vi "U01_8_5 ReadExcelActiveX.vi"(8 "error in (no error)":errorcluster, 10 "NameSheet":string, 11 "References":T1) -> (0 "error out":errorcluster, 2 "data":string[][](array[string]), 3 "References":T1)   [LabVIEW 2019]
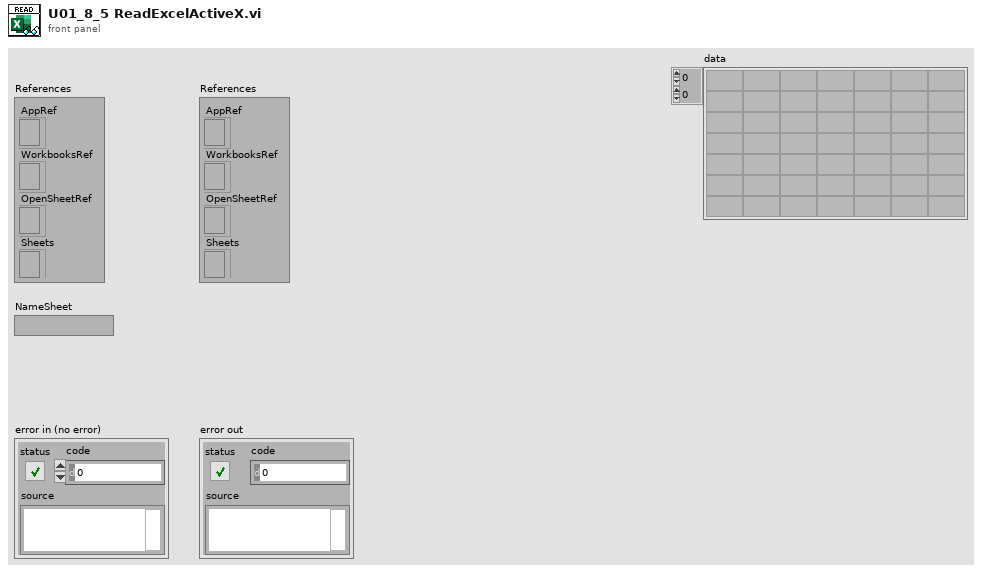
[diagram p1: front panel]
types:
  T1 = cluster{"AppRef":refnum<k7>, "WorkbooksRef":refnum<k7>, "OpenSheetRef":refnum<k7>, "Sheets":refnum<k7>}
  T2 = cluster{"AppRef":refnum<k7>, "WorkbooksRef":refnum<k7>, "OpenSheetRef":refnum<k7>, "Excel._Worksheet":refnum<k7>}
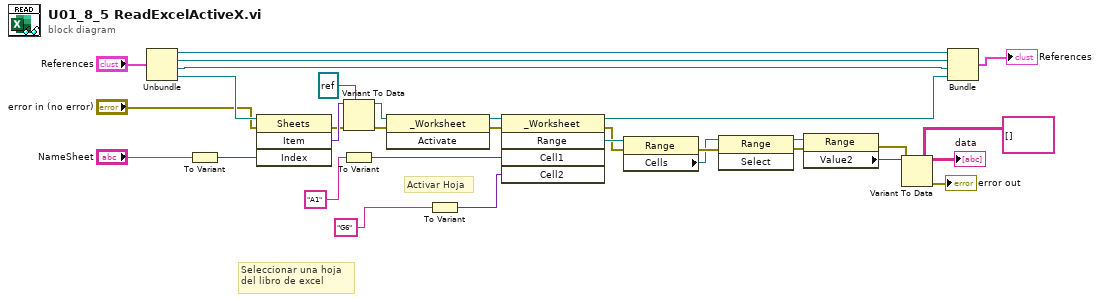
[diagram p0: block diagram]
diagram:
  # "Activar Hoja"
  # "Seleccionar una hoja \ndel libro de excel"
  n1 = Unbundle("References") -> ("AppRef"=w17:refnum<k7>, "WorkbooksRef"=w16:refnum<k7>, "OpenSheetRef"=w6:refnum<k7>, "Sheets"=w31:refnum<k7>)
  n2 = To Variant(anything="NameSheet") -> (Variant=w25:variant)
  n3 = invoke class="Sheets" method="Item"(reference=w31, error in="error in (no error)", "Index"=w25) -> (error out=w19:errorcluster, "Item"=w28:variant)  [unwired: 1 in, 2 out]
  n4 = Variant To Data(error in=w19, type=refnum<k7> refnum ("Excel._Worksheet"), Variant=w28) -> (data=w20:refnum<k7>, error out=w21:errorcluster)
  n5 = To Variant(anything="A1") -> (Variant=w27:variant)
  n6 = invoke class="_Worksheet" method="Activate"(reference=w20, error in=w21) -> (reference out=w24:refnum<k7>, error out=w22:errorcluster)  [unwired: 1 in, 1 out]
  n7 = To Variant(anything="G6") -> (Variant=w23:variant)
  n8 = invoke class="_Worksheet" method="Range"(reference=w24, error in=w22, "Cell1"=w27, "Cell2"=w23) -> (reference out=w15:refnum<k7>, error out=w12:errorcluster, "Range"=w13:refnum<k7>)  [unwired: 1 in, 2 out]
  n9 = property class="Range"(reference=w13, error in=w12) -> (error out=w11:errorcluster, "Cells"=w10:refnum<k7>)  [unwired: 1 out]
  n10 = invoke class="Range" method="Select"(reference=w10, error in=w11) -> (reference out=w7:refnum<k7>, error out=w8:errorcluster)  [unwired: 1 in, 1 out]
  n11 = property class="Range"(reference=w7, error in=w8) -> (error out=w5:errorcluster, "Value2"=w4:variant)  [unwired: 1 out]
  n12 = Variant To Data(error in=w5, type=string[][] [], Variant=w4) -> (data=→"data":string[][], error out=→"error out":errorcluster)
  n13 = Bundle("AppRef"=w17, "WorkbooksRef"=w16, "OpenSheetRef"=w6, "Excel._Worksheet"=w15) -> (→"References":T2)  [unwired: 1 in]
